vi "Test Customer Update Order Number Broadcasts Order Number.vi"(8 "error in (no error)":errorcluster, 11 "Customer Test in":refnum<class "Customer Test.lvclass">) -> (0 "error out":errorcluster, 3 "Customer Test out":refnum<class "Customer Test.lvclass">)   [LabVIEW 2020, in "Customer Test.lvclass"]
uses:
  Customer Test.lvclass
  C:/Program Files (x86)/National Instruments/LabVIEW 2020/vi.lib/Asteme/LUnit/Test Case.lvclass
  Customer/Customer.lvclass
  C:/Program Files (x86)/National Instruments/LabVIEW 2020/vi.lib/Asteme/Triarc Framework/Process/Process.lvclass
  Customer/Private/Order State.ctl
  <vilib>/Asteme/Triarc Framework/Process/Process.lvclass/Process.ctl
  <vilib>/Asteme/LUnit/Test Case.lvclass/Test Case.ctl
  <vilib>/Asteme/LUnit/LUnit Assertion Result.lvclass/LUnit Assertion Result.ctl
  <vilib>/Asteme/Triarc Framework Test Suite/Support/Execution timer.vi
  <vilib>/Asteme/Triarc Framework/Process/Private/SubVIs/Wait for finish.vi
  <vilib>/Asteme/Triarc Framework/Process/Protected/Messaging/Enqueue Message.vi
  <vilib>/Asteme/Triarc Framework/Process/Private/SubVIs/Set Lifecycle State.vi
  <vilib>/Asteme/Triarc Framework/Process/Public/Lifecycle/Get Lifecycle State.vi
  <vilib>/Asteme/LUnit/Palette/Pass.vi
  <vilib>/Asteme/LUnit/Palette/Fail.vi
  <vilib>/Asteme/LUnit/Variant to string.vi
  <vilib>/Asteme/LUnit/Set Assertion Type.vi
  <vilib>/AdvancedString/1D String Array to Delimited String.vi
  <vilib>/Utility/error.llb/Clear Errors.vi
  <vilib>/Asteme/LUnit/Add test result.vi
  <vilib>/Asteme/LUnit/LUnit Write Passed.vi
  <vilib>/Asteme/LUnit/LUnit Get Test Case.vi
  <vilib>/Asteme/LUnit/Assertion Result/LUnit Get Test Name.vi
  <vilib>/Asteme/LUnit/LUnit Write Message.vi
  <vilib>/Asteme/LUnit/LUnit Write Description.vi
  <vilib>/Asteme/LUnit/LUnit Write Assertion Type.vi
  <vilib>/Asteme/LUnit/Read Test Case Name.vi
  <vilib>/Asteme/Triarc Framework Test Suite/Support/Event Helpers/Dequeue Event Message.vi
  <vilib>/Utility/error.llb/Error Cluster From Error Code.vi
  <vilib>/Utility/Data Type/Get Type Information.vi
  <vilib>/Utility/LVClass/Get LV Class Name.vi
  <vilib>/Asteme/LUnit/LUnit Assertion Result.lvclass
  <vilib>/Asteme/Triarc Framework/Process/Process.lvclass
  <vilib>/Asteme/Triarc Framework Test Suite/Support/Event Helpers/Event Helpers.lvlib
  <vilib>/Asteme/LUnit/Test Case.lvclass
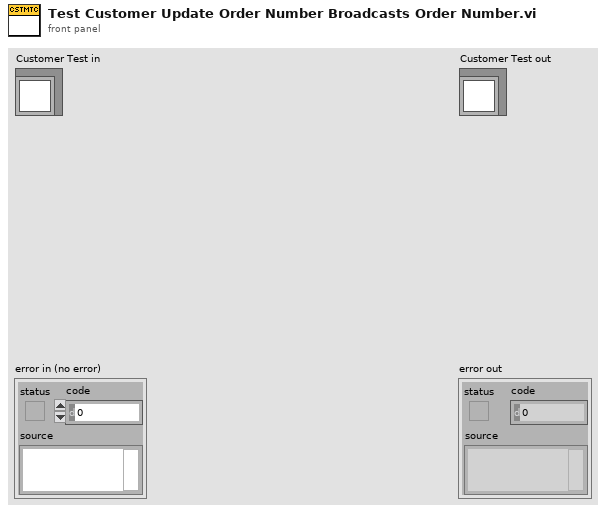
[diagram p1: front panel]
types:
  T1 = typedef "Customer.lvclass/Order State.ctl" = cluster{"Order In Progress?":bool, "Order Number":u32, "Order Price":dbl, "Items Ordered":u32, "Items Received":u32, "Items Picked Up":string}
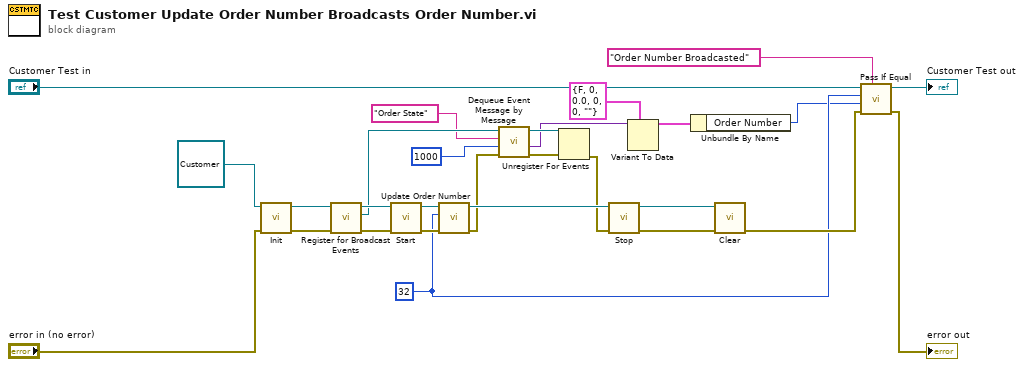
[diagram p0: block diagram]
diagram:
  w5 = u32 32 ("Order Number")
  n1 = call-dynamic "Init.vi"("error in (no error)"="error in (no error)", "View In"=refnum<class "Customer.lvclass"> refnum ("Customer.lvclass")) -> ("error out"=w24:errorcluster, "View Out"=w25:refnum<class "Customer.lvclass">)  [unwired: 8 in]
  n2 = call <vilib>:"Register for Broadcast Events.vi"("error in (no error)"=w24, "Process In"=w25) -> ("error out"=w27:errorcluster, "Event Registration Refnum Out"=w20:refnum<event-registration>, "Process Out"=w26:refnum<class "Customer.lvclass">)  [unwired: 7 in]
  n3 = call <vilib>:"Start.vi"("error in (no error)"=w27, "Process In"=w26) -> ("error out"=w17:errorcluster, "Process Out"=w19:refnum<class "Customer.lvclass">)  [unwired: 8 in]
  n4 = call "Update Order Number.vi"("error in (no error)"=w17, "Order Number"=w5, "Customer In"=w19) -> ("error out"=w16:errorcluster, "Customer Out"=w18:refnum<class "Customer.lvclass">)  [unwired: 7 in]
  n5 = call <vilib>:"Dequeue Event Message by Message.vi"("error in (no error)"=w16, "Timeout (-1)"=1000, "Message"="Order State", "Event Registration Refnum"=w20) -> ("error out"=w15:errorcluster, "Message Data"=w2:variant, "Event Registration Refnum Out"=w8:refnum<event-registration>)  [unwired: 3 in, 2 out]
  n6 = Unregister For Events(event registration refnum=w8, error in=w15) -> (error out=w12:errorcluster)
  n7 = call <vilib>:"Stop.vi"("error in (no error)"=w12, "Process In"=w18) -> ("error out"=w22:errorcluster, "Process Out"=w23:refnum<class "Customer.lvclass">)  [unwired: 7 in, 1 out]
  n8 = Variant To Data(type=T1 {"Order In Progress?"=FALSE, "Order Number"=0, "Order Price"=0.0, "Items Ordered"=0, "Items Received"=0, "Items Picked Up"=""} ("Order State"), Variant=w2) -> (data=w3:T1)  [unwired: 1 in, 1 out]
  n9 = Unbundle By Name(w3) -> ("Order Number"=w1:u32)
  n10 = call-dynamic "Clear.vi"("error in (no error)"=w22, "View In"=w23) -> ("error out"=w11:errorcluster)  [unwired: 9 in]
  n11 = call <vilib>:"Pass If Equal.vi"("Description"="Order Number Broadcasted", "error in (no error)"=w11, "Actual"=w1, "Expected"=w5, "Test Case In"="Customer Test in") -> ("error out"=→"error out":errorcluster, "Test Case Out"=→"Customer Test out":refnum<class "Customer Test.lvclass">)  [unwired: 5 in]
